vi "norm unknown cycle simple.vi"(9 "output cluster 2":T1 {"cycle results dbl" format="%#_11f"}) -> (1 "output cluster":T1 {"cycle results dbl" format="%#_11f"})   [LabVIEW 2016]
uses:
  controls/cycle results control.ctl
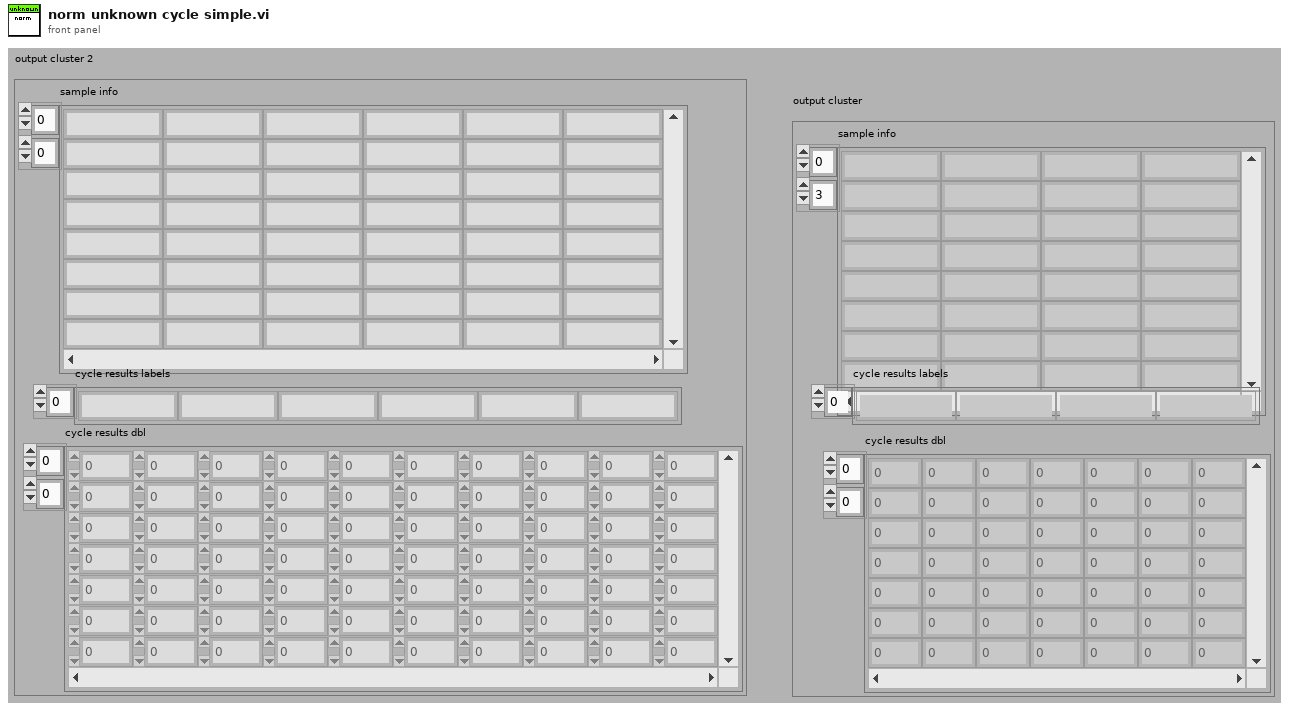
[diagram p1: front panel]
types:
  T1 = typedef "cycle results control.ctl" = cluster{"sample info":string[][], "cycle results labels":string[], "cycle results dbl":dbl[][]}
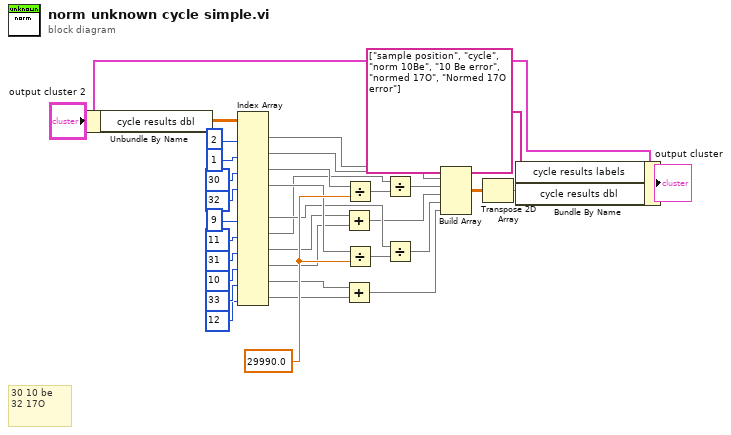
[diagram p0: block diagram]
diagram:
  w30 = 29990.0 ("y")
  # "30 10 be\n32 17O"
  n1 = Unbundle By Name("output cluster 2") -> ("cycle results dbl"=w33:dbl[][])
  n2 = Index Array(array=w33, index (col) #1=2 ("disabled index (col)"), index (col) #2=1 ("disabled index (col)"), index (col) #3=30 ("disabled index (col)"), index (col) #4=32 ("index (col)"), index (col) #6=9 ("index (col)"), index (col) #7=11 ("index (col)"), index (col) #8=31 ("index (col)"), index (col) #9=10 ("index (col)"), index (col) #10=33 ("index (col)"), index (col) #11=12 ("index (col)")) -> (element #1=w1:dbl[], element #2=w12:dbl[], element #3=w28:dbl[], element #4=w29:dbl[], element #6=w24:dbl[], element #7=w22:dbl[], element #8=w19:dbl[], element #9=w18:dbl[], element #10=w14:dbl[], element #11=w15:dbl[])  [unwired: 12 in, 1 out]
  n3 = Add(x=w19, y=w18) -> (x+y=w10:dbl[])
  n4 = Add(x=w14, y=w15) -> (x+y=w8:dbl[])
  n5 = Divide(x=w28, y=w30) -> (x/y=w23:dbl[])
  n6 = Divide(x=w29, y=w30) -> (x/y=w25:dbl[])
  n7 = Divide(x=w22, y=w23) -> (x/y=w11:dbl[])
  n8 = Divide(x=w24, y=w25) -> (x/y=w9:dbl[])
  n9 = Build Array(w1, w12, w11, w10, w9, w8) -> (w4:dbl[][])
  n10 = Transpose 2D Array(2D array=w4) -> (transposed array=w3:dbl[][])
  n11 = Bundle By Name(cluster="output cluster 2", "cycle results labels"=string[] ["sample position", "cycle", "norm 10Be", "10 Be error", "normed 17O", "Normed 17O error"], "cycle results dbl"=w3) -> (→"output cluster":T1)
